vi "基础10.vi"() -> ()   [LabVIEW 2014]
panel:
  out "输出变量":dbl
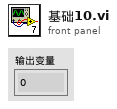
[diagram p1: front panel]
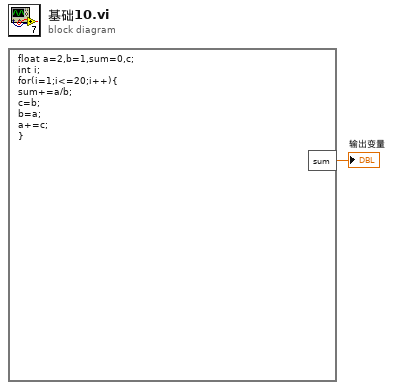
[diagram p0: block diagram]
diagram:
  n1 = formula code="float a=2,b=1,sum=0,c;\nint i;\nfor(i=1;i<=20;i++){\nsum+=a/b;\nc=b;\nb=a;\na+=c;\n}"() -> ("sum"=→"输出变量":dbl)
